vi "VMUIselfTerminateTest.vi"() -> ()   [LabVIEW 2013]
uses:
  VariableManagerCodes/VariableManager/VariableManager.lvclass
  VariableManagerCodes/API/VariableManagerAPI.lvlib
panel:
  in  "Stop":bool
  in  "Start":bool
  in  "VariableManagerTest":refnum<class "VariableManager.lvclass">
  # "1. Run and click \"Start VMUI\"\n    Do step 1 multiple times will open multiple UI\n    for the same VariableManager database\n   (The database is the \"VariableManagerTest\" object in this window)\n2. On the VMUI window(s), try click \"Stop Client\"\n    while VMUI still attach to client's subpanel.\n3. Wait for 10seconds to see VMUI detach itself from the closed client.\n4. Close this window will make reference to database invalid.\n    Try close this window and see VMUI close itself in 10 seconds."
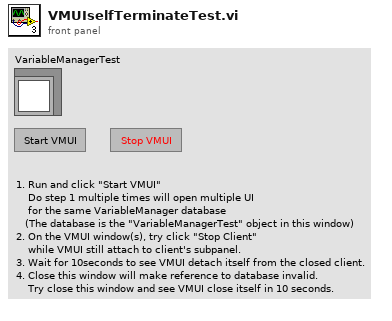
[diagram p1: front panel]
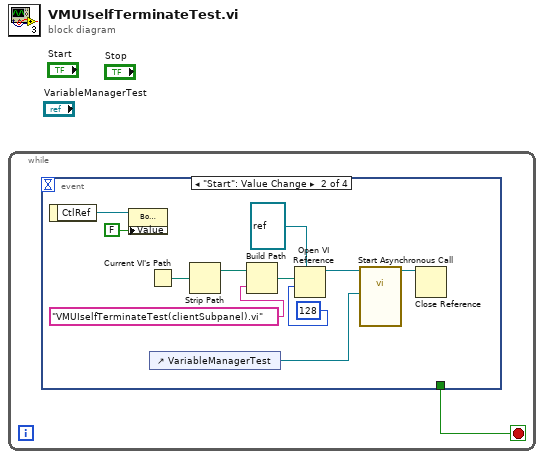
[diagram p0: block diagram]
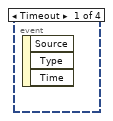
[diagram p2: hidden frame]
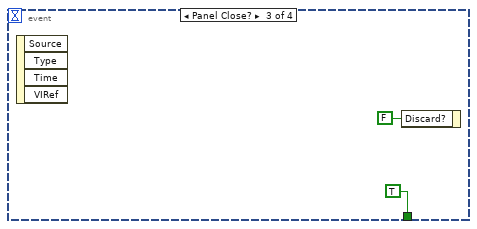
[diagram p3: hidden frame]
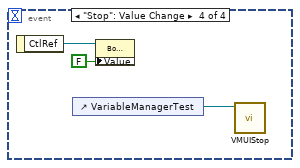
[diagram p4: hidden frame]
diagram:
  n1 = while {
    stop <- w1 stop-if-true
    n2 = event shown="[1] \"Start\": Value Change" {
      selector: _ -> [_ _ _ _]
      dyn-events: _ -> [_ _ _ _]
      timeout: _ -> [_ _ _ _]
      tunnel: [_ _ TRUE _] -> w1
      event Timeout {
        n3 = event-data() -> ()  [unwired: 1 in, 3 out]
      }
      event "Start": Value Change {
        n4 = event-data() -> ("CtlRef"=w11:refnum<vi>)  [unwired: 1 in]
        n5 = property class="Bool (strict)"(reference=w11, "Value"=FALSE) -> ()  [unwired: 1 in, 2 out]
        n6 = Current VI's Path() -> (path=w6:path)
        n7 = control-ref of="VariableManagerTest"() -> (w3:refnum<vi>)
        n8 = Strip Path(path=w6) -> (stripped path=w5:path)  [unwired: 1 out]
        n9 = Build Path(base path=w5, name or relative path="VMUIselfTerminateTest(clientSubpanel).vi") -> (appended path=w7:path)
        n10 = Open VI Reference(type specifier VI Refnum (for type only)=refnum<vi> refnum, vi path=w7, options=128) -> (vi reference=w9:refnum<vi>)  [unwired: 3 in, 1 out]
        n11 = call-by-ref "Start Asynchronous Call"(reference=w9, "VariableManagerRef in"=w3) -> (reference out=w2:refnum<vi>)  [unwired: 12 in, 1 out]
        n12 = Close Reference(reference=w2) -> ()  [unwired: 1 in, 1 out]
      }
      event Panel Close? {
        n13 = event-data() -> ()  [unwired: 1 in, 4 out]
        n14 = event-data("Discard?"=FALSE) -> ()  [unwired: 1 in, 1 out]
      }
      event "Stop": Value Change {
        n15 = event-data() -> ("CtlRef"=w16:refnum<vi>)  [unwired: 1 in]
        n16 = control-ref of="VariableManagerTest"() -> (w15:refnum<vi>)
        n17 = property class="Bool (strict)"(reference=w16, "Value"=FALSE) -> ()  [unwired: 1 in, 2 out]
        n18 = call "VMUIStop.vi"("VariableManagerRef in"=w15) -> ()  [unwired: 9 in, 2 out]
      }
    }
  }
